vi "Insert Turns.vi"(1 "Sideways Turn Movement":i32, 2 "Forward Turn Movement":i32, 3 "Merged Instructions":i32[][](array[numeric])) -> (0 "Instructions":i32[][](array[numeric]))   [LabVIEW 2015]
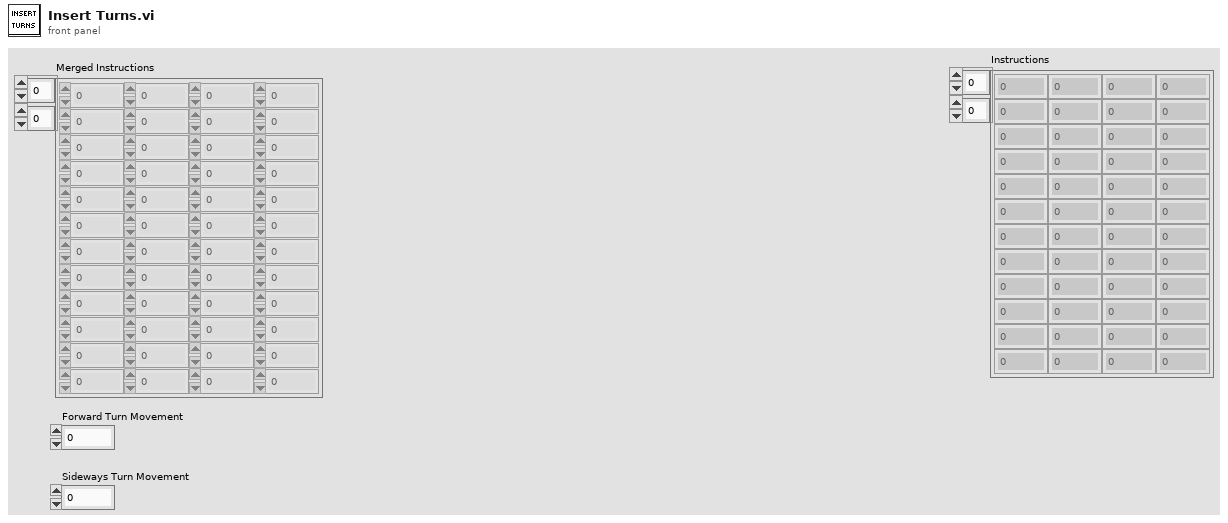
[diagram p1: front panel]
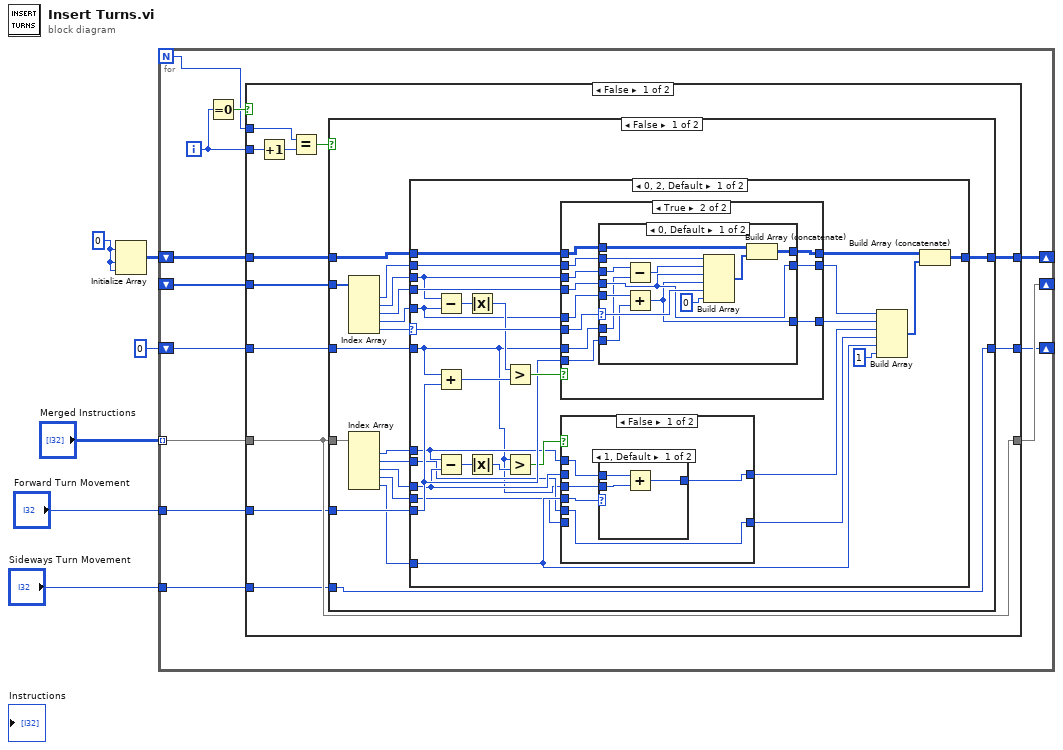
[diagram p0: block diagram]
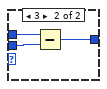
[diagram p2: hidden frame]
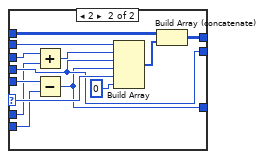
[diagram p5: hidden frame]
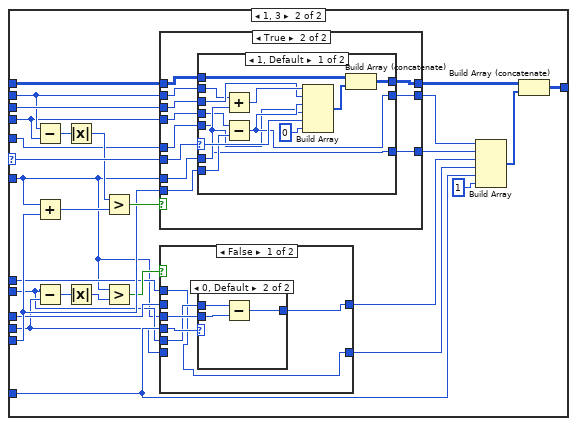
[diagram p6: hidden frame]
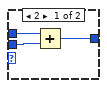
[diagram p7: hidden frame]
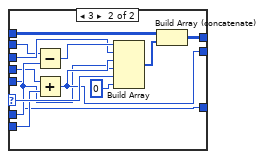
[diagram p10: hidden frame]
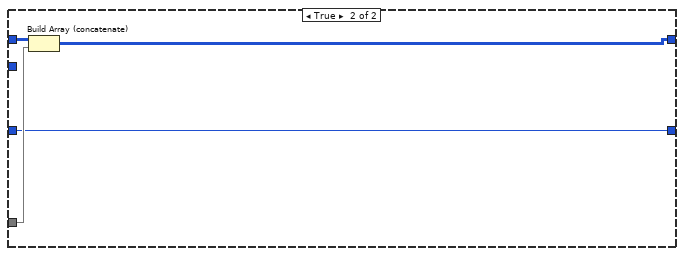
[diagram p11: hidden frame]
diagram:
  w6 = 0
  n1 = Initialize Array(w6, w6, w6) -> (w5:i32[][])
  n2 = for {
    N -> [w11]
    shift-right: [w17] -> _
    shift-left: w5 -> [w16]
    shift-right: [w15] -> _
    shift-left: _ -> [w13]
    tunnel: "Merged Instructions" -> [w14] mode=indexing
    tunnel: "Forward Turn Movement" -> [w10]
    shift-right: [w8] -> _
    shift-left: 0 -> [w9]
    tunnel: "Sideways Turn Movement" -> [w7]
    i -> [w12]
    n3 = Equal To 0?(x=w12) -> (x = 0?=w18:bool)
    n4 = case shown="False" w18 {
      tunnel: [w23 w216] -> w17
      tunnel: w16 -> [w24 w216]
      tunnel: [w29 w215] -> w15
      tunnel: w14 -> [w29 w215]
      tunnel: w13 -> [w30 _]
      tunnel: w12 -> [w27 _]
      tunnel: w11 -> [w26 _]
      tunnel: w10 -> [w22 _]
      tunnel: w9 -> [w21 w214]
      tunnel: [w20 w214] -> w8
      tunnel: w7 -> [w19 _]
      frame False {
        n5 = Increment(x=w27) -> (x+1=w28:i32)
        n6 = Equal?(x=w26, y=w28) -> (x = y?=w25:bool)
        n7 = case shown="False" w25 {
          tunnel: w30 -> [w47 _]
          tunnel: w29 -> [w46 w213]
          tunnel: w24 -> [w42 w212]
          tunnel: [w38 w211] -> w23
          tunnel: w22 -> [w39 _]
          tunnel: w21 -> [w37 w210]
          tunnel: [w36 w210] -> w20
          tunnel: w19 -> [w36 _]
          frame False {
            n8 = Index Array(array=w47) -> (element #1=w44:i32, element #2=w41:i32, element #3=w43:i32, element #4=w40:i32, element #5=w45:i32)  [unwired: 5 in]
            n9 = Index Array(array=w46) -> (element #1=w34:i32, element #2=w31:i32, element #3=w33:i32, element #4=w32:i32, element #5=w35:i32)  [unwired: 5 in]
            n10 = case shown="0, 2, Default" w45 {
              selector: w45 -> [w73 w154]
              tunnel: w44 -> [w71 w133]
              tunnel: w43 -> [w70 w132]
              tunnel: w42 -> [w72 w153]
              tunnel: w41 -> [w59 w142]
              tunnel: w40 -> [w58 w141]
              tunnel: w39 -> [w60 w143]
              tunnel: [w66 w149] -> w38
              tunnel: w37 -> [w48 w129]
              tunnel: w35 -> [w61 w144]
              tunnel: w34 -> [w51 w135]
              tunnel: w33 -> [w50 w134]
              tunnel: w32 -> [w53 w131]
              tunnel: w31 -> [w49 w130]
              frame 0, 2, Default {
                n11 = Subtract(x=w59, y=w58) -> (x-y=w75:i32)
                n12 = Add(x=w48, y=w60) -> (x+y=w68:i32)
                n13 = Subtract(x=w51, y=w50) -> (x-y=w57:i32)
                n14 = Absolute Value(x=w75) -> (abs(x)=w69:i32)
                n15 = Absolute Value(x=w57) -> (abs(x)=w56:i32)
                n16 = Greater?(x=w69, y=w68) -> (0:w74:bool)
                n17 = Greater?(x=w48, y=w56) -> (0:w55:bool)
                n18 = case shown="True" w74 {
                  tunnel: w73 -> [_ w102]
                  tunnel: w72 -> [w91 w101]
                  tunnel: w71 -> [w89 w100]
                  tunnel: w59 -> [w90 w99]
                  tunnel: w58 -> [_ w98]
                  tunnel: w70 -> [_ w97]
                  tunnel: [w91 w96] -> w67
                  tunnel: w60 -> [_ w95]
                  tunnel: [w90 w94] -> w63
                  tunnel: [w89 w93] -> w64
                  tunnel: w48 -> [_ w92]
                  frame False {
                  }
                  frame True {
                    n19 = case shown="0, Default" w102 {
                      selector: w102 -> [w113 w126]
                      tunnel: w101 -> [w115 w128]
                      tunnel: w100 -> [w114 w127]
                      tunnel: w99 -> [w105 w118]
                      tunnel: w98 -> [w107 w120]
                      tunnel: w97 -> [w108 w121]
                      tunnel: w95 -> [w109 w122]
                      tunnel: [w110 w123] -> w96
                      tunnel: [w106 w119] -> w94
                      tunnel: [w108 w121] -> w93
                      tunnel: w92 -> [w104 w117]
                      frame 0, Default {
                        n20 = Subtract(x=w105, y=w104) -> (x-y=w103:i32)
                        n21 = Add(x=w107, y=w109) -> (x+y=w106:i32)
                        n22 = Build Array(w114, w103, w108, w106, w113, 0 ("element")) -> (w111:i32[])
                        n23 = Build Array (concatenate)(w115, w111) -> (w110:i32[][])
                      }
                      frame 2 {
                        n24 = Add(x=w118, y=w117) -> (x+y=w116:i32)
                        n25 = Subtract(x=w120, y=w122) -> (x-y=w119:i32)
                        n26 = Build Array(w127, w116, w121, w119, w126, 0 ("element")) -> (w124:i32[])
                        n27 = Build Array (concatenate)(w128, w124) -> (w123:i32[][])
                      }
                    }
                  }
                }
                n28 = case shown="False" w55 {
                  tunnel: w61 -> [w80 _]
                  tunnel: w50 -> [_ w88]
                  tunnel: [w77 w88] -> w54
                  tunnel: w53 -> [_ w87]
                  tunnel: [w76 w87] -> w52
                  tunnel: w51 -> [w79 _]
                  tunnel: w48 -> [w78 _]
                  tunnel: w49 -> [w76 _]
                  frame False {
                    n29 = case shown="1, Default" w80 {
                      tunnel: w79 -> [w83 w86]
                      tunnel: w78 -> [w82 w85]
                      tunnel: [w81 w84] -> w77
                      frame 1, Default {
                        n30 = Add(x=w83, y=w82) -> (x+y=w81:i32)
                      }
                      frame 3 {
                        n31 = Subtract(x=w86, y=w85) -> (x-y=w84:i32)
                      }
                    }
                  }
                  frame True {
                  }
                }
                n32 = Build Array(w64, w63, w54, w52, w61, 1) -> (w62:i32[])
                n33 = Build Array (concatenate)(w67, w62) -> (w66:i32[][])
              }
              frame 1, 3 {
                n34 = Subtract(x=w133, y=w132) -> (x-y=w156:i32)
                n35 = Add(x=w129, y=w143) -> (x+y=w151:i32)
                n36 = Subtract(x=w130, y=w131) -> (x-y=w140:i32)
                n37 = Absolute Value(x=w156) -> (abs(x)=w152:i32)
                n38 = Absolute Value(x=w140) -> (abs(x)=w139:i32)
                n39 = Greater?(x=w152, y=w151) -> (0:w155:bool)
                n40 = Greater?(x=w129, y=w139) -> (0:w138:bool)
                n41 = case shown="True" w155 {
                  tunnel: w154 -> [_ w183]
                  tunnel: w153 -> [w172 w182]
                  tunnel: w133 -> [w170 w181]
                  tunnel: w142 -> [w171 w180]
                  tunnel: w141 -> [_ w179]
                  tunnel: w132 -> [_ w178]
                  tunnel: [w172 w177] -> w150
                  tunnel: w143 -> [_ w176]
                  tunnel: [w171 w175] -> w146
                  tunnel: [w170 w174] -> w147
                  tunnel: w129 -> [_ w173]
                  frame False {
                  }
                  frame True {
                    n42 = case shown="1, Default" w183 {
                      selector: w183 -> [w195 w208]
                      tunnel: w182 -> [w196 w209]
                      tunnel: w181 -> [w187 w200]
                      tunnel: w180 -> [w188 w201]
                      tunnel: w179 -> [w184 w197]
                      tunnel: w178 -> [w186 w199]
                      tunnel: w176 -> [w191 w204]
                      tunnel: [w192 w205] -> w177
                      tunnel: [w184 w197] -> w175
                      tunnel: [w185 w198] -> w174
                      tunnel: w173 -> [w190 w203]
                      frame 1, Default {
                        n43 = Add(x=w187, y=w190) -> (x+y=w189:i32)
                        n44 = Subtract(x=w186, y=w191) -> (x-y=w185:i32)
                        n45 = Build Array(w189, w188, w185, w184, w195, 0 ("element")) -> (w193:i32[])
                        n46 = Build Array (concatenate)(w196, w193) -> (w192:i32[][])
                      }
                      frame 3 {
                        n47 = Subtract(x=w200, y=w203) -> (x-y=w202:i32)
                        n48 = Add(x=w199, y=w204) -> (x+y=w198:i32)
                        n49 = Build Array(w202, w201, w198, w197, w208, 0 ("element")) -> (w206:i32[])
                        n50 = Build Array (concatenate)(w209, w206) -> (w205:i32[][])
                      }
                    }
                  }
                }
                n51 = case shown="False" w138 {
                  tunnel: w144 -> [w161 _]
                  tunnel: w134 -> [_ w169]
                  tunnel: [w159 w169] -> w137
                  tunnel: w131 -> [_ w168]
                  tunnel: [w157 w168] -> w136
                  tunnel: w135 -> [w157 _]
                  tunnel: w129 -> [w160 _]
                  tunnel: w130 -> [w158 _]
                  frame False {
                    n52 = case shown="0, Default" w161 {
                      tunnel: w158 -> [w164 w167]
                      tunnel: w160 -> [w163 w166]
                      tunnel: [w162 w165] -> w159
                      frame 2 {
                        n53 = Add(x=w164, y=w163) -> (x+y=w162:i32)
                      }
                      frame 0, Default {
                        n54 = Subtract(x=w167, y=w166) -> (x-y=w165:i32)
                      }
                    }
                  }
                  frame True {
                  }
                }
                n55 = Build Array(w147, w146, w137, w136, w144, 1) -> (w145:i32[])
                n56 = Build Array (concatenate)(w150, w145) -> (w149:i32[][])
              }
            }
          }
          frame True {
            n57 = Build Array (concatenate)(w212, w213) -> (w211:i32[][])
          }
        }
      }
      frame True {
      }
    }
  }
